vi "Close.vi"(8 "error in (no error)":errorcluster, 11 "PS Driver AMI4xx Actor in":refnum<class "PS Driver AMI4xx.lvclass">) -> (0 "error out":errorcluster, 3 "PS Driver AMI4xx Actor out":refnum<class "PS Driver AMI4xx.lvclass">)   [LabVIEW 2019, in "PS Driver.lvlib" / "PS Driver AMI4xx.lvclass"]
uses:
  PS Driver AMI4xx.lvclass
  Users/Shared/NML Data Acquisition/SCM PS Actor Framework/PS Driver/PS Driver.lvclass
  PS Driver.lvclass/PS Driver.ctl
  PS Driver with Persistence.lvclass
  PS Driver.lvclass
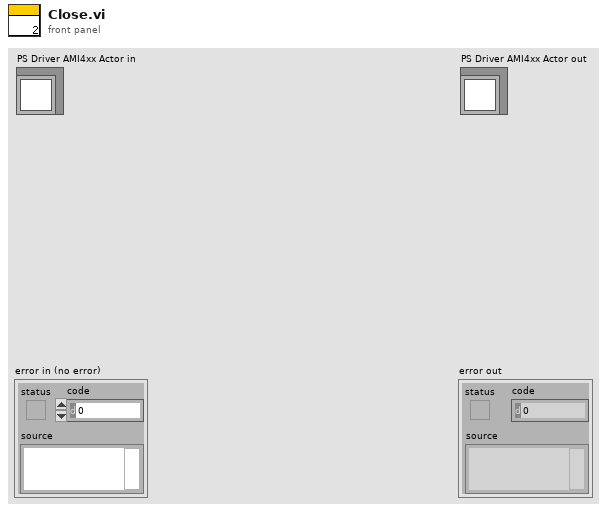
[diagram p1: front panel]
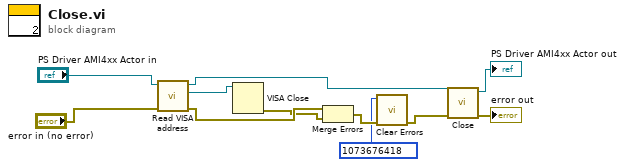
[diagram p0: block diagram]
diagram:
  n1 = call "Read VISA address.vi"("error in (no error)"="error in (no error)", "PS Driver in"="PS Driver AMI4xx Actor in") -> ("error out"=w5:errorcluster, "VISA address"=w9:refnum<visa-resource-name>, "PS Driver out"=w8:refnum<class "PS Driver AMI4xx.lvclass">)  [unwired: 7 in]
  n2 = VISA Close(VISA resource name=w9) -> (error out=w4:errorcluster)  [unwired: 1 in]
  n3 = Merge Errors(w5, w4) -> (w3:errorcluster)
  n4 = call <vilib>:"Clear Errors.vi"("error in (no error)"=w3, "specific error code to clear (0: all)"=1073676418) -> ("error out"=w1:errorcluster)  [unwired: 4 in, 1 out]
  n5 = call-parent "Close.vi"("error in (no error)"=w1, "PS Driver Actor in"=w8) -> ("error out"=→"error out":errorcluster, "PS Driver Actor out"=→"PS Driver AMI4xx Actor out":refnum<class "PS Driver AMI4xx.lvclass">)  [unwired: 8 in]
